vi "Creat XLS by Station.vi"(2 "staiton":T2, 3 "data in":string[](array[string]), 4 "2D data":string[][](array[string]) caption="二维数据") -> (6 "new file path (Not A Path if cancelled)":path caption="新建文件路径（取消时为非法路径）")   [LabVIEW 2014]
uses:
  DefCtrl/Station.ctl
  DefCtrl/ListInf.ctl
panel:
  in  "List Inf":T1={"粗切工位"=["生产时间", "料车号", "切割文件", "最大光强", "最小光强", "切割速度", "生产节拍", "产量", "项目类型", "过程条码"], "热处理工位"=["生产时间", "料车号", "加热开始时间", "加热结束时间", "设定加热时长", "实际加热时长", "设定加热温度", "项目类型", "过程条码"], "精切工位"=["生产时间", "上料料车号", "切割文件", "最大光强", "最小光强", "切割速度", "生产节拍", "产量", "项目类型", "下料料车号", "过程条码"], "PDF工位"={"List 1"=["生产时间", "料车号", "项目类型", "过程条码", "振幅（%）", "滑台速度", "焊接滑台位置", "压型滑台位置", "焊接开始时间", "焊接结束时间"], "List 2"=["压型进口温度1", "压型进口温度2", "压型进口温度3", "压型进口温度4", "压型进口温度5", "压型进口温度6", "压型进口温度7", "压型进口温度8", "压型进口温度9", "压型进口温度10", "压型进口温度11", "压型进口温度12", "压型进口温度13", "压型进口温度14", "压型进口温度15", "压型进口温度16", "压型进口温度17", "压型进口温度18", "压型进口温度19", "压型进口温度20", "压型进口温度21", "压型进口温度22", "压型进口温度23", "压型进口温度24", "压型进口温度25", "压型进口温度26", "压型进口温度27", "压型进口温度28", "压型进口温度29", "压型进口温度30"], "List 3"=["焊接出口温度1", "焊接出口温度2", "焊接出口温度3", "焊接出口温度4", "焊接出口温度5", "焊接出口温度6", "焊接出口温度7", "焊接出口温度8", "焊接出口温度9", "焊接出口温度10", "焊接出口温度11", "焊接出口温度12", "焊接出口温度13", "焊接出口温度14", "焊接出口温度15", "焊接出口温度16", "焊接出口温度17", "焊接出口温度18", "焊接出口温度19", "焊接出口温度20", "焊接出口温度21", "焊接出口温度22", "焊接出口温度23", "焊接出口温度24", "焊接出口温度25", "焊接出口温度26", "焊接出口温度27", "焊接出口温度28", "焊接出口温度29", "焊接出口温度30"], "List 4"=["压力值1", "压力值2", "压力值3", "压力值4", "压力值5", "压力值6", "压力值7", "压力值8", "压力值9", "压力值10", "压力值11", "压力值12", "压力值13", "压力值14", "压力值15", "压力值16", "压力值17", "压力值18", "压力值19", "压力值20", "压力值21", "压力值22", "压力值23", "压力值24", "压力值25", "压力值26", "压力值27", "压力值28", "压力值29", "压力值30"]}, "打凹点工位"=["生产时间", "扭矩值", "圈数", "当前项目"], "检测工位"=["流水号", "时间", "收回1力值", "收回2力值", "收回3力值", "收回4力值", "展开1力值", "展开2力值", "展开3力值", "展开4力值", "项目号", "Pass/Fail"]}
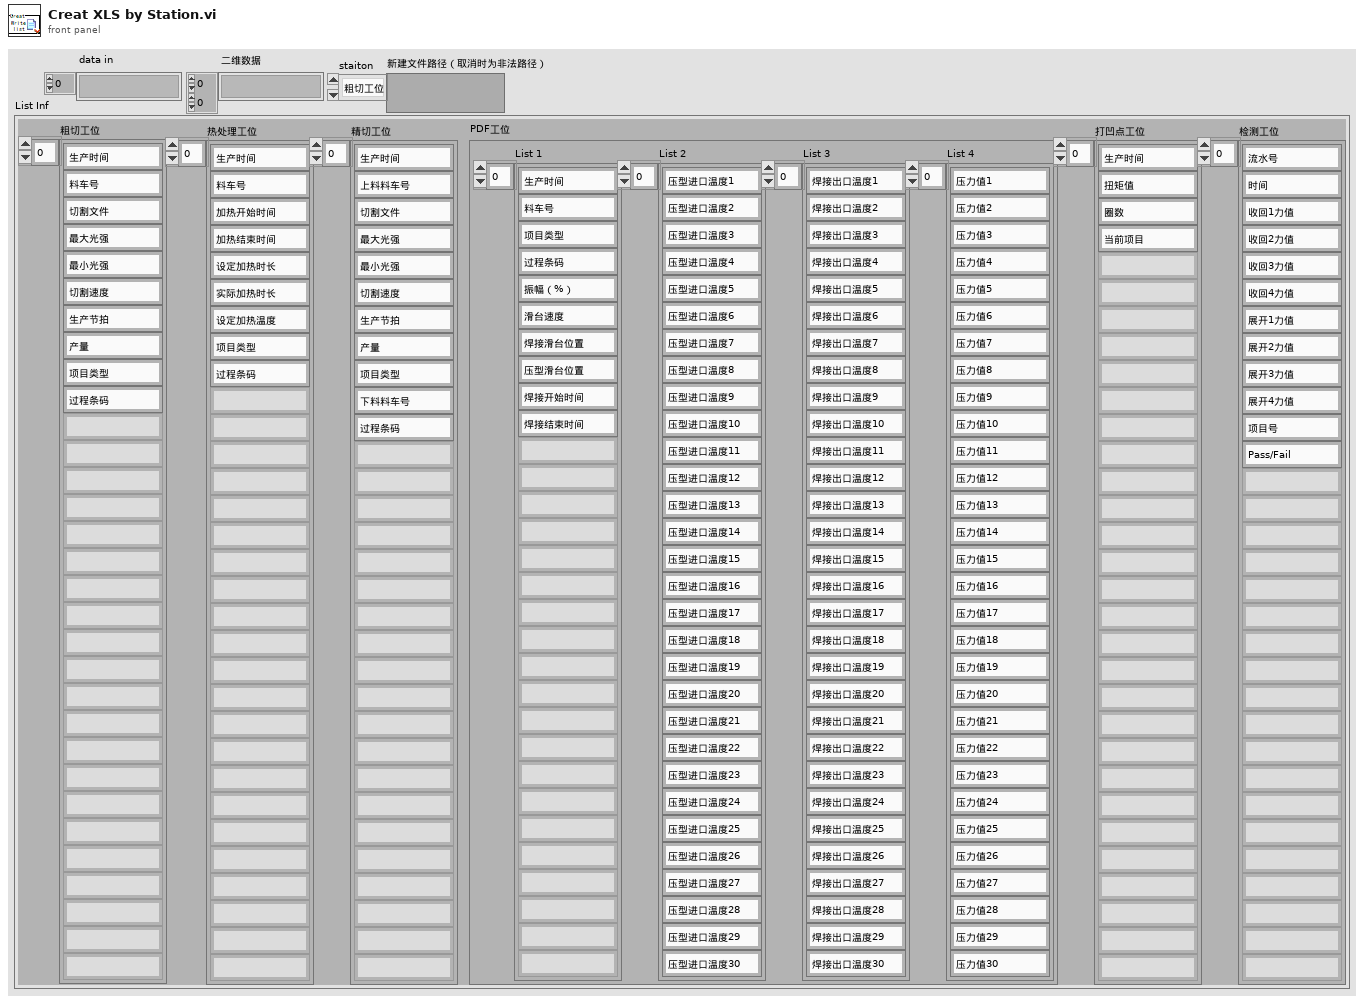
[diagram p1: front panel]
types:
  T1 = typedef "ListInf.ctl" = cluster{"粗切工位":string[], "热处理工位":string[], "精切工位":string[], "PDF工位":cluster{"List 1":string[], "List 2":string[], "List 3":string[], "List 4":string[]}, "打凹点工位":string[], "检测工位":string[]}
  T2 = typedef "Station.ctl" = enum16{"粗切工位", "热处理工位", "精切工位", "PDF焊接工位", "打凹点预载力工位", "收卷工位", "EOL工位"}
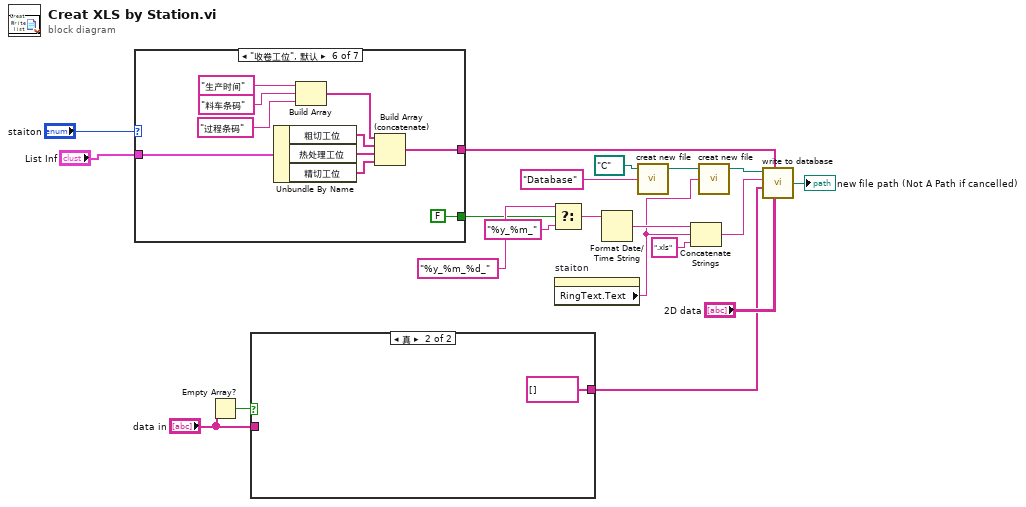
[diagram p0: block diagram]
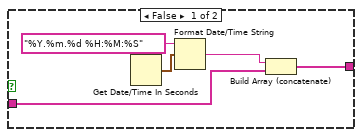
[diagram p2: hidden frame]
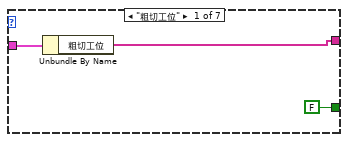
[diagram p3: hidden frame]
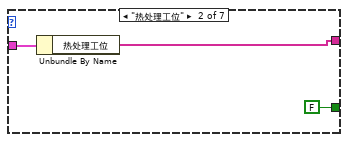
[diagram p4: hidden frame]
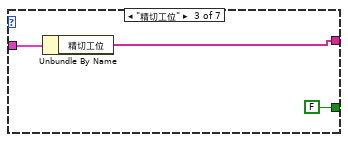
[diagram p5: hidden frame]
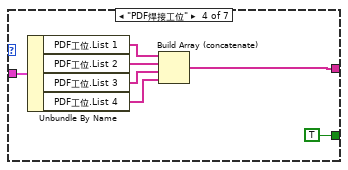
[diagram p6: hidden frame]
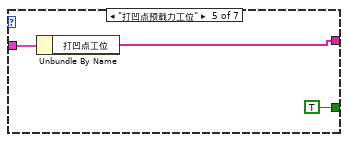
[diagram p7: hidden frame]
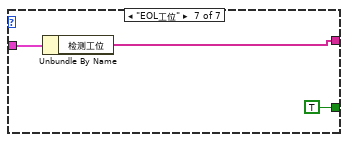
[diagram p8: hidden frame]
diagram:
  n1 = case shown="\"收卷工位\", 默认" "staiton" {
    tunnel: [w22 w25 w28 w31 w38 w49 w51] -> w8
    tunnel: [FALSE FALSE FALSE TRUE TRUE FALSE TRUE] -> w6
    tunnel: "List Inf" -> [w21 w24 w27 w30 w37 w41 w50]
    frame "粗切工位" {
      n2 = Unbundle By Name(w21) -> ("粗切工位"=w22:string[])
    }
    frame "热处理工位" {
      n3 = Unbundle By Name(w24) -> ("热处理工位"=w25:string[])
    }
    frame "精切工位" {
      n4 = Unbundle By Name(w27) -> ("精切工位"=w28:string[])
    }
    frame "PDF焊接工位" {
      n5 = Unbundle By Name(w30) -> ("PDF工位.List 1"=w35:string[], "PDF工位.List 2"=w34:string[], "PDF工位.List 3"=w33:string[], "PDF工位.List 4"=w32:string[])
      n6 = Build Array (concatenate)(w35, w34, w33, w32) -> (w31:string[])
    }
    frame "打凹点预载力工位" {
      n7 = Unbundle By Name(w37) -> ("打凹点工位"=w38:string[])
    }
    frame "收卷工位", Default {
      n8 = Unbundle By Name(w41) -> ("粗切工位"=w47:string[], "热处理工位"=w46:string[], "精切工位"=w45:string[])
      n9 = Build Array("生产时间", "料车条码", "过程条码") -> (w42:string[])
      n10 = Build Array (concatenate)(w42, w47, w46, w45) -> (w49:string[])
    }
    frame "EOL工位" {
      n11 = Unbundle By Name(w50) -> ("检测工位"=w51:string[])
    }
  }
  n12 = Empty Array?(array="data in") -> (empty?=w2:bool)
  n13 = case shown="真" w2 {
    tunnel: [w54 string[] []] -> w4
    tunnel: "data in" -> [w53 _]
    frame False {
      n14 = Get Date/Time In Seconds() -> (seconds since 1Jan1904=w57:timestamp)
      n15 = Format Date/Time String(time format string (%c)="%Y.%m.%d %H:%M:%S" ("时间格式字符串(%c)"), seconds (now)=w57) -> (date/time string=w55:string)  [unwired: 1 in]
      n16 = Build Array (concatenate)(w55, w53) -> (w54:string[])
    }
    frame True {
    }
  }
  n17 = Select(t="%y_%m_%d_" ("时间格式字符串(%c)"), s=w6, f="%y_%m_" ("时间格式字符串(%c)")) -> (s? t:f=w13:string)
  n18 = property on="staiton" class="Enum (严格)"() -> ("RingText.Text"=w5:string)  [unwired: 2 in, 2 out]
  n19 = Format Date/Time String(time format string (%c)=w13) -> (date/time string=w18:string)  [unwired: 2 in]
  n20 = call "creat new file.vi"("file name"="Database", "path"=path "C:/") -> ("created path"=w15:path)  [unwired: 1 in, 2 out]
  n21 = Concatenate Strings(w18, w5, ".xls" ("字符串")) -> (w16:string)
  n22 = call "creat new file.vi"("file name"=w5, "path"=w15) -> ("created path"=w14:path)  [unwired: 1 in, 2 out]
  n23 = call "write to database.vi"("2D data"="2D data", "Header"=w8, "data in"=w4, "file name"=w16, "path"=w14) -> ("new file path (Not A Path if cancelled)"=→"new file path (Not A Path if cancelled)":path)  [unwired: 1 in]
